vi "Solve Center Wavelength v0.52.vi"(4 "Standard Wavelength":dbl=500.0 format="%.2f", 6 "Current Central Wavelength":dbl=600.0 format="%.2f", 7 "pixel index":dbl=200.0 min=0.0 max=1024.0 format="%.2f", 8 "Current Grating Density":enum16{"150", "300", "600", "1200", "1800"}(ring)=enum."600" caption="Grating Density") -> (3 "Calibrated Central Wavelength":dbl=517.6607981427933 format="%.4f")   [LabVIEW 2024]
panel:
  out "Final Difference":dbl=2.3305801732931286e-12 format="%.2e"
  out "Iterations needed":i32=4
  in  "Maximum Iterations":u16=1000
  out "Current Wavelength":dbl=582.5031806844609 format="%.4f"
  in  "Tolerance":dbl=1e-10 format="%.2e"
  out "Calculated Standard Wavelength":dbl=499.99999999999767 format="%.4f"
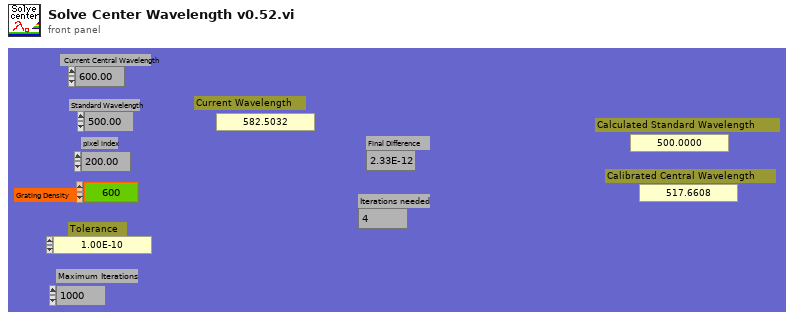
[diagram p1: front panel]
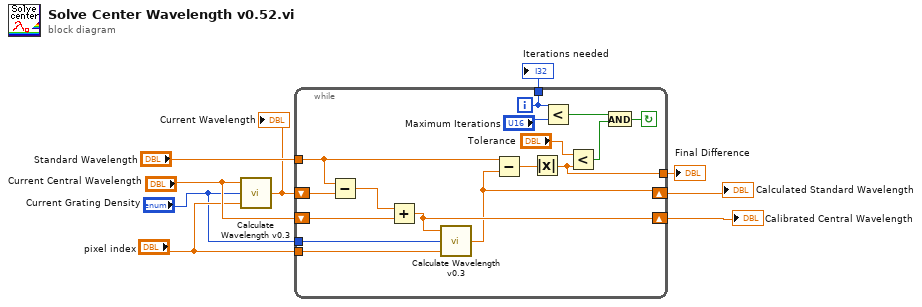
[diagram p0: block diagram]
diagram:
  n1 = call "Calculate Wavelength v0.3.vi"("pixel index"="pixel index", "Current Grating Density"="Current Grating Density", "Central Wavelength"="Current Central Wavelength") -> ("nm (out)"=w3:dbl)  [unwired: 2 in]
  "Current Wavelength" <- w3
  n2 = while {
    tunnel: [w10] -> w1
    tunnel: [w11] -> w2
    tunnel: "Standard Wavelength" -> [w19]
    shift-left: "Current Central Wavelength" -> [w24]
    shift-right: [w21] -> w7
    tunnel: "pixel index" -> [w22]
    tunnel: "Current Grating Density" -> [w23]
    shift-left: w3 -> [w25]
    shift-right: [w18] -> w8
    i -> [w11]
    stop <- w14 continue-if-true
    n3 = Subtract(x=w19, y=w25) -> (x-y=w20:dbl)
    n4 = Add(x=w20, y=w24) -> (x+y=w21:dbl)
    n5 = call "Calculate Wavelength v0.3.vi"("pixel index"=w22, "Current Grating Density"=w23, "Central Wavelength"=w21) -> ("nm (out)"=w18:dbl)  [unwired: 2 in]
    n6 = Subtract(x=w19, y=w18) -> (x-y=w17:dbl)
    n7 = Absolute Value(x=w17) -> (abs(x)=w10:dbl)
    n8 = Less?(x=w11, y="Maximum Iterations") -> (x < y?=w13:bool)
    n9 = Less?(x="Tolerance", y=w10) -> (x < y?=w12:bool)
    n10 = And(x=w13, y=w12) -> (x .and. y?=w14:bool)
  }
  "Calibrated Central Wavelength" <- w7
  "Calculated Standard Wavelength" <- w8
  "Iterations needed" <- w2
  "Final Difference" <- w1
